vi "nominal client new.vi"(7 "out_client":i32, 8 "error in (no error)":errorcluster, 9 "base_url":string, 10 "workspace_rid":string, 11 "token":string) -> (0 "error out":errorcluster, 3 "function return":i32, 5 "out_client out":i32)   [LabVIEW 2020, in "client.lvlib"]
doc: "int32_t nominal_client_new(const char *token,\n const char *workspace_rid,\n const char *base_url,\n int32_t *out_client);"
uses:
  client.lvlib
  nominalClient_64.dll
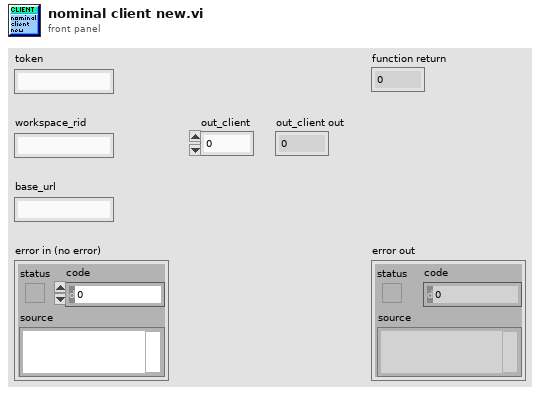
[diagram p1: front panel]
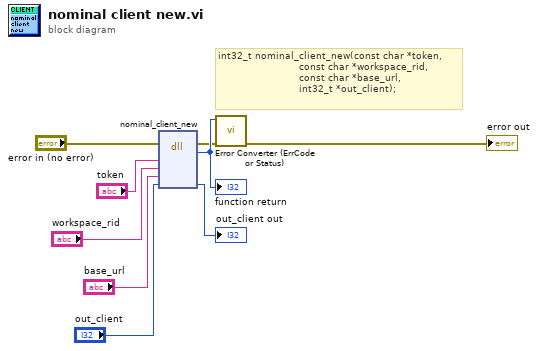
[diagram p0: block diagram]
diagram:
  # "int32_t nominal_client_new(const char *token,\n                           const char *workspace_rid,\n                           const char *base_url,\n                           int32_t *out_client);"
  n1 = dll-call lib="C:/code/labview-client-rs/lv_src/client/nominalClient_*.*" fn="nominal_client_new"(error in="error in (no error)", "token"="token", "workspace_rid"="workspace_rid", "base_url"="base_url", "out_client"="out_client") -> (error out=w2:errorcluster, w9:i32, "out_client"=→"out_client out":i32)  [unwired: 5 in, 1 out]
  "function return" <- w9
  n2 = call "Error Converter (ErrCode or Status).vi"("error in (no error)"=w2, "error code"=w9) -> ("error out"=→"error out":errorcluster)  [unwired: 9 in]
